vi "Test_OSC_v3.vi"() -> ()   [LabVIEW 2010]
uses:
  <instrlib>/niScope/Controls/niScope trigger slope.ctl
  <instrlib>/niScope/Controls/niScope trigger coupling.ctl
  <instrlib>/niScope/Controls/niScope vertical coupling.ctl
  <vilib>/Utility/error.llb/DialogType.ctl
  <instrlib>/niScope/Controls/niScope timestamp type.ctl
  <instrlib>/niScope/Configure/Trigger/niScope Configure Trigger Edge.vi
  <vilib>/Waveform/WDTFileIO.llb/Export Waveforms To Spreadsheet File (1D).vi
panel:
  in  "file path (dialog if empty)":path=path "D:/GSSor/Test_OSC/LOGS"
  out "error out":errorcluster {"code" format="%.0x"}
  in  "channel name":string="0" caption="Channel Name(s)"
  in  "enforce realtime":bool=TRUE caption="Enforce Realtime"
  in  "vertical range":dbl=10.0 caption="Vertical Range (V)" format="%.2f"
  in  "min sample rate":dbl=250000000.0 caption="Min. Sample Rate" step=1000000.0 format="%.2p"
  in  "min record length":i32=100 caption="Min. Record Length"
  out "Waveform Graph":waveform(dbl)[](graph)
  in  "timeout (s)":dbl=-1.0 caption="Timeout(s)" format="%.2f"
  in  "vertical offset":dbl caption="Vertical Offset" format="%.4f"
  in  "probe attenuation":dbl=10.0 caption="Probe Attenuation" format="%.1f"
  in  "input impedance":u32(ring) caption="Input Impedance" items=["1 mega ohm"=0, "50 ohms"=2]
  in  "maximum input frequency":dbl=250.0 caption="Max. Input Frequency" format="%.2p"
  in  "trigger delay":dbl caption="Trigger Delay" format="%.4p"
  in  "reference position":dbl=50.0 caption="Ref Position" format="%.1f"
  in  "trigger level":dbl=0.1 caption="Trigger Level" format="%.2f"
  in  "stop":bool
  in  "vertical coupling":T1=1 caption="Vertical Coupling" items=["AC", "DC", "Ground"]
  in  "trigger coupling":T2=1 caption="Trigger Coupling" items=["AC"=0, "DC"=1, "HF Reject"=3, "LF Reject"=4, "AC Plus HF Reject"=1001]
  in  "trigger slope":T3 caption="Trigger Slope"
  in  "trigger source":string(combo)="0" caption="Trigger Source"
  in  "trigger modifier":i32(ring)=1 caption="Trigger Modifier" items=["None"=1, "Auto Trigger"=2]
  in  "resource name":refnum<k15>="PXI1Slot5" caption="Resource Name"
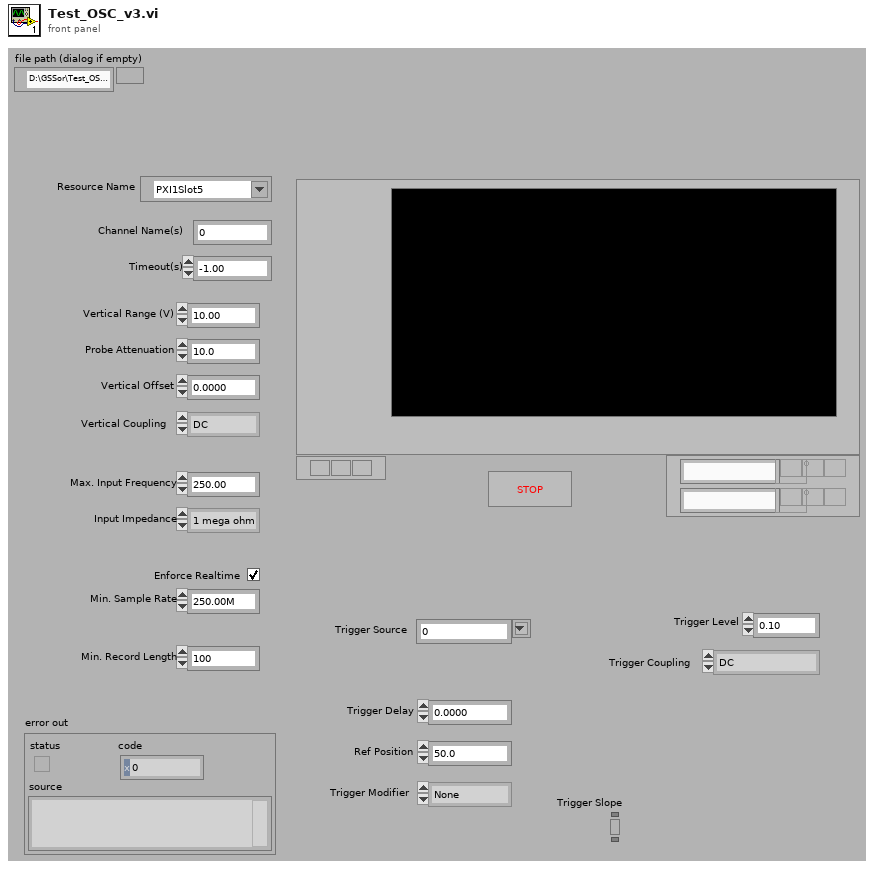
[diagram p1: front panel]
types:
  T1 = typedef "niScope vertical coupling.ctl" = i32
  T2 = typedef "niScope trigger coupling.ctl" = u16
  T3 = typedef "niScope trigger slope.ctl" = i32
  T4 = typedef "DialogType.ctl" = u16
  T5 = typedef "niScope timestamp type.ctl" = i32
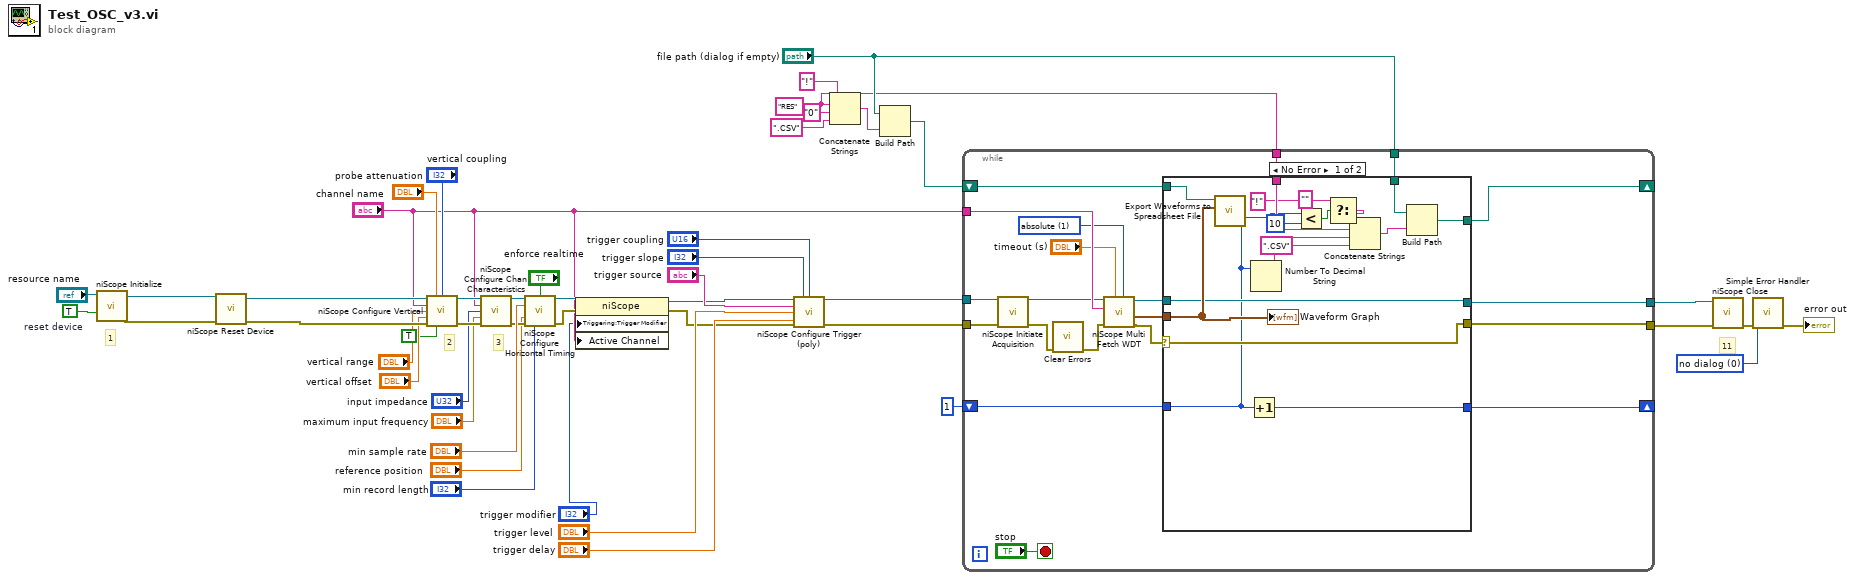
[diagram p0: block diagram]
diagram:
  w4 = "RES" ("string")
  w12 = T4 0 items=["no dialog", "OK message", "continue or stop message", "OK message + warnings", "continue/stop + warnings"] ("type of dialog (OK msg:1)")
  w47 = TRUE  # reset device
  # "2"
  # "3"
  # "11"
  # "1"
  n1 = call <instrlib>:"niScope Initialize.vi"("resource name"="resource name", "reset device"=w47) -> ("instrument handle"=w40:refnum<k15>, "error out"=w41:errorcluster)  [unwired: 12 in]
  n2 = call <instrlib>:"niScope Reset Device.vi"("instrument handle"=w40, "error in"=w41) -> ("instrument handle out"=w42:refnum<k15>, "error out"=w43:errorcluster)  [unwired: 12 in]
  n3 = call <instrlib>:"niScope Configure Vertical.vi"("instrument handle"=w42, "probe attenuation"="probe attenuation", "vertical coupling"="vertical coupling", "channels"="channel name", "vertical range"="vertical range", "vertical offset"="vertical offset", "error in"=w43, "channel enabled"=TRUE) -> ("instrument handle out"=w36:refnum<k15>, "error out"=w35:errorcluster)  [unwired: 6 in]
  n4 = call <instrlib>:"niScope Configure Chan Characteristics.vi"("instrument handle"=w36, "channels"="channel name", "input impedance"="input impedance", "maximum input frequency"="maximum input frequency", "error in"=w35) -> ("instrument handle out"=w33:refnum<k15>, "error out"=w34:errorcluster)  [unwired: 9 in]
  n5 = call <instrlib>:"niScope Configure Horizontal Timing.vi"("instrument handle"=w33, "enforce realtime"="enforce realtime", "min sample rate"="min sample rate", "reference position"="reference position", "error in"=w34, "min record length"="min record length") -> ("instrument handle out"=w21:refnum<k15>, "error out"=w20:errorcluster)  [unwired: 8 in]
  n6 = property class="niScope"(reference=w21, error in=w20, "Triggering:Trigger Modifier"="trigger modifier", "Active Channel"="channel name") -> (reference out=w18:refnum<k15>, error out=w19:errorcluster)
  n7 = call-poly <instrlib>:"niScope Configure Trigger (poly).vi"("instrument handle"=w18, "trigger slope"="trigger slope", "trigger coupling"="trigger coupling", "trigger source"="trigger source", "trigger level"="trigger level", "error in"=w19, "trigger delay"="trigger delay") -> ("instrument handle out"=w10:refnum<k15>, "error out"=w9:errorcluster)  [unwired: 7 in]
  n8 = Concatenate Strings("!" ("string"), w4, "0" ("string"), ".CSV" ("string")) -> (w6:string)
  n9 = Build Path(base path="file path (dialog if empty)", name or relative path=w6) -> (appended path=w5:path)
  n10 = while {
    tunnel: "channel name" -> [w67]
    tunnel: [w53] -> w8
    tunnel: [w54] -> w13
    shift-right: [w59] -> _
    shift-left: w5 -> [w65]
    tunnel: "file path (dialog if empty)" -> [w63]
    tunnel: w4 -> [w62]
    shift-right: [w60] -> _
    shift-left: 1 -> [w61]
    tunnel: w10 -> [w57]
    tunnel: w9 -> [w56]
    stop <- "stop" stop-if-true
    w51 = T5 1 items=["relative", "absolute"] ("timestamp Type")
    n11 = call <instrlib>:"niScope Initiate Acquisition.vi"("instrument handle"=w57, "error in"=w56) -> ("instrument handle out"=w48:refnum<k15>, "error out"=w49:errorcluster)  [unwired: 12 in]
    n12 = call <vilib>:"Clear Errors.vi"("error in (no error)"=w49) -> ("error out"=w50:errorcluster)  [unwired: 6 in]
    n13 = call "niScope Multi Fetch WDT.vi"("timestamp Type"=w51, "timeout"="timeout (s)", "error in"=w50, "channels"=w67, "instrument handle"=w48) -> ("error out"=w58:errorcluster, "wfm"=w64:waveform(dbl)[], "instrument handle out"=w55:refnum<k15>)  [unwired: 3 in, 1 out]
    n14 = case shown="No Error" w58 {
      selector: w58 -> [w76 w85]
      tunnel: w65 -> [w84 w88]
      tunnel: w64 -> [w83 _]
      tunnel: w63 -> [w82 _]
      tunnel: w62 -> [w81 _]
      tunnel: w61 -> [w73 w87]
      tunnel: [w78 w87] -> w60
      tunnel: [w77 w88] -> w59
      tunnel: w55 -> [w75 w86]
      tunnel: [w75 w86] -> w54
      tunnel: [w76 w85] -> w53
      frame No Error {
        n15 = call-poly <vilib>:"Export Waveforms to Spreadsheet File.vi"("waveforms"=w83, "file path (dialog if empty)"=w84) -> ()  [unwired: 8 in, 2 out]
        n16 = Increment(x=w73) -> (x+1=w78:i32)
        n17 = Number To Decimal String(number=w73) -> (decimal integer string=w80:string)  [unwired: 1 in]
        n18 = Less?(x=w73, y=10) -> (x < y?=w71:bool)
        n19 = Select(t="!" ("string"), s=w71, f="") -> (s? t:f=w69:string)
        n20 = Concatenate Strings(w69, w81, w80, ".CSV" ("string")) -> (w79:string)
        n21 = Build Path(base path=w82, name or relative path=w79) -> (appended path=w77:path)
        "Waveform Graph" <- w83
      }
      frame Error {
      }
    }
  }
  n22 = call <instrlib>:"niScope Close.vi"("instrument handle"=w13, "error in"=w8) -> ("error out"=w45:errorcluster)  [unwired: 13 in]
  n23 = call <vilib>:"Simple Error Handler.vi"("type of dialog (OK msg:1)"=w12, "error in (no error)"=w45) -> ("error out"=→"error out":errorcluster)  [unwired: 3 in, 4 out]
